vi "AIT 429 - Load Database.vi"(8 "error in (no error)":errorcluster, 11 "Node Ptr":u64 format="%.0x") -> (0 "error out":errorcluster)   [LabVIEW 2012, in "AIT 429 System Explorer.lvlib"]
uses:
  AIT 429 System Explorer.lvlib
  SubVIs/Create Sysdef Tree from DB Channel Clusters.vi
  SubVIs/Create Sysdef Tree Labels.vi
  SubVIs/Build Label Properties.vi
  Shared/Controls and Global/Global.vi
  <vilib>/NI Veristand/Custom Device API/Get Item Property (Path).vi
  SubVIs/Parse DB/Parse DB.vi
  <vilib>/NI Veristand/Custom Device API/NI VeriStand - Enable System Explorer Update Buffer.vi
  <vilib>/NI Veristand/Custom Device Tools/Custom Device Utility Library/NI VeriStand - Search for Item.vi
  <vilib>/NI Veristand/Custom Device Tools/Custom Device Utility Library/NI VeriStand - Search for Item by GUID.vi
  <vilib>/NI Veristand/Custom Device API/NI VeriStand - Add Custom Device Section.vi
  <vilib>/NI Veristand/Custom Device API/NI VeriStand - Add Custom Device Channel.vi
  SubVIs/AddParamChannels.vi
  <vilib>/NI Veristand/Custom Device API/NI VeriStand - Commit System Explorer Update Buffer.vi
  <vilib>/NI Veristand/Custom Device API/Set Item Property (String).vi
  <vilib>/NI Veristand/Custom Device API/Set Item Property (Path).vi
  <vilib>/NI Veristand/Custom Device API/Custom Device API.lvlib
  ARINC 429 Shared.lvlib
  <vilib>/NI Veristand/Custom Device Tools/Custom Device Utility Library/Custom Device Utility Library.lvlib
panel:
  in  "Tag":string
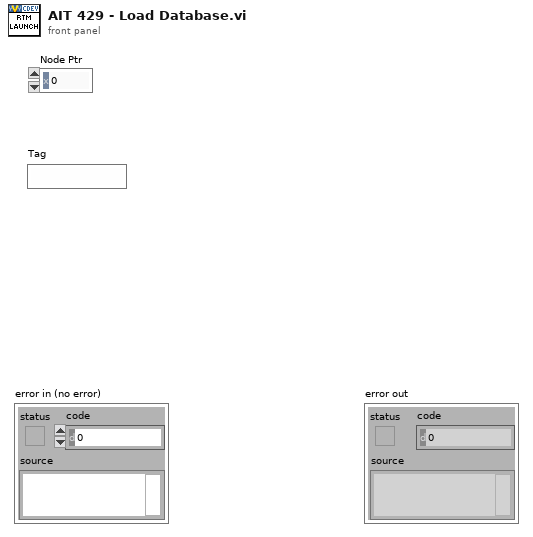
[diagram p1: front panel]
types:
  T1 = typedef "Custom Device API.lvlib/Custom Device Item Ref.ctl" = u64
  T2 = typedef "AIT 429 System Explorer.lvlib/Refresh Match Settings.ctl" = cluster{"Ch by name?":bool, "Lbl by name?":bool}
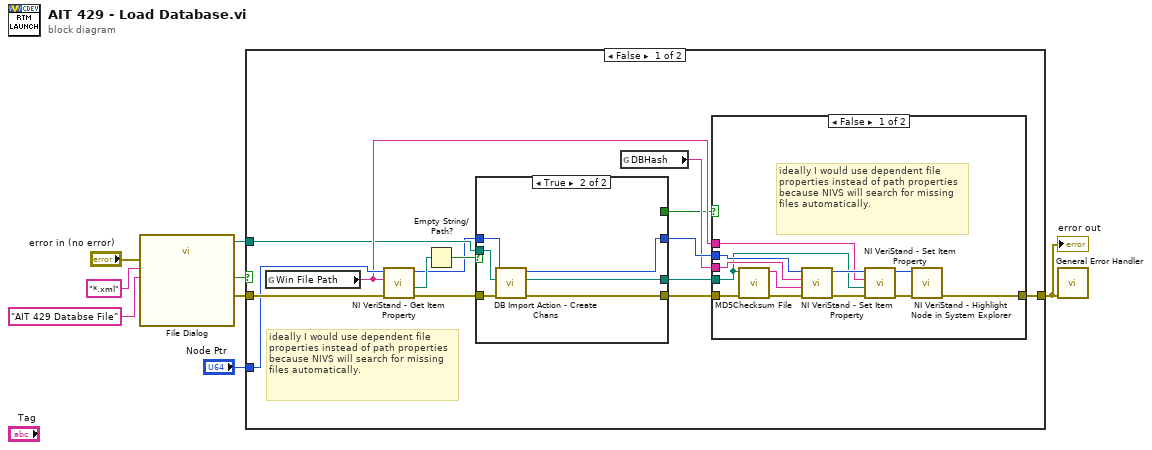
[diagram p0: block diagram]
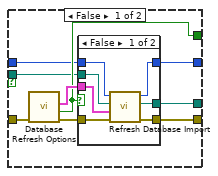
[diagram p3: hidden frame]
diagram:
  n1 = call "File Dialog"("error in"="error in (no error)", "pattern (all files)"="*.xml", "pattern label"="AIT 429 Databse File") -> ("selected path"=w1:path, "cancelled"=w4:bool, "error out"=w3:errorcluster)  [unwired: 9 in, 1 out]
  n2 = case shown="False" w4 {
    tunnel: [w19 w61] -> w8
    tunnel: w3 -> [w17 w61]
    tunnel: "Node Ptr" -> [w16 _]
    tunnel: w1 -> [w12 _]
    frame False {
      # "ideally I would use dependent file properties instead of path properties because NIVS will search for missing files automatically."
      n3 = global read "Global.vi" "Win File Path"() -> (w15:string)
      n4 = call-poly <vilib>:"NI VeriStand - Get Item Property.vi"("error in (no error)"=w17, "Property Name"=w15, "Item Ref in"=w16) -> ("error out"=w9:errorcluster, "Value"=w13:path, "Item Ref out"=w10:T1)  [unwired: 5 in, 1 out]
      n5 = Empty String/Path?(string/path=w13) -> (empty?=w11:bool)
      n6 = case shown="True" w11 {
        tunnel: [w42 w60] -> w22
        tunnel: [w41 w59] -> w21
        tunnel: [w39 w58] -> w20
        tunnel: w9 -> [w44 w57]
        tunnel: [w38 _] -> w14
        tunnel: w12 -> [w37 w56]
        tunnel: w10 -> [w36 w55]
        frame False {
          n7 = call "Database Refresh Options.vi"("error in (no error)"=w44) -> ("error out"=w43:errorcluster, "Cancelled?"=w38:bool, "Refresh Settings"=w40:T2)  [unwired: 8 in]
          n8 = case shown="False" w38 {
            tunnel: w43 -> [w51 w54]
            tunnel: [w50 w54] -> w42
            tunnel: [w49 w52] -> w41
            tunnel: w37 -> [w46 w53]
            tunnel: w40 -> [w48 _]
            tunnel: [w47 w53] -> w39
            tunnel: w36 -> [w45 w52]
            frame False {
              n9 = call "Refresh Database Import.vi"("error in (no error)"=w51, "Match settings"=w48, "DB"=w46, "Item Ref in"=w45) -> ("error out"=w50:errorcluster, "DB dup"=w47:path, "Item Ref dup"=w49:T1)  [unwired: 5 in]
            }
            frame True {
            }
          }
        }
        frame True {
          n10 = call "DB Import Action - Create Chans.vi"("error in (no error)"=w57, "selected path"=w56, "Node Ptr"=w55) -> ("error out"=w60:errorcluster, "selected path out"=w58:path, "Node Ptr dup"=w59:u64)  [unwired: 6 in]
        }
      }
      n11 = global read "Global.vi" "DBHash"() -> (w18:string)
      n12 = case shown="False" w14 {
        tunnel: w22 -> [w26 w35]
        tunnel: w21 -> [w34 _]
        tunnel: w20 -> [w23 _]
        tunnel: [w33 w35] -> w19
        tunnel: w18 -> [w28 _]
        tunnel: w15 -> [w27 _]
        frame False {
          # "ideally I would use dependent file properties instead of path properties because NIVS will search for missing files automatically."
          n13 = call <vilib>:"MD5Checksum File.vi"("error in (no error)"=w26, "Path"=w23) -> ("error out"=w25:errorcluster, "MD5 message-digest"=w24:string)  [unwired: 8 in]
          n14 = call-poly <vilib>:"NI VeriStand - Set Item Property.vi"("error in (no error)"=w25, "Value"=w24, "Property Name"=w28, "Item Ref in"=w34) -> ("error out"=w29:errorcluster, "Item Ref out"=w30:T1)  [unwired: 5 in, 1 out]
          n15 = call-poly <vilib>:"NI VeriStand - Set Item Property.vi"("error in (no error)"=w29, "Value"=w23, "Property Name"=w27, "Item Ref in"=w30) -> ("error out"=w32:errorcluster, "Item Ref out"=w31:T1)  [unwired: 5 in, 1 out]
          n16 = call <vilib>:"NI VeriStand - Highlight Node in System Explorer.vi"("error in (no error)"=w32, "Item Ref in"=w31) -> ("error out"=w33:errorcluster)  [unwired: 8 in, 1 out]
        }
        frame True {
        }
      }
    }
    frame True {
    }
  }
  "error out" <- w8
  n17 = call <vilib>:"General Error Handler.vi"("error in (no error)"=w8) -> ()  [unwired: 10 in, 5 out]
